vi "Write Coils.vi"(8 "error in (no error)":errorcluster, 9 "values":bool[](array[boolean]), 10 "address":i32, 11 "modbus in":refnum<class "libmodbus.lvclass">) -> (0 "error out":errorcluster, 3 "modbus out":refnum<class "libmodbus.lvclass">)   [LabVIEW 2017, in "libmodbus.lvlib" / "libmodbus.lvclass"]
doc: "Writes single modbus holding register."
uses:
  libmodbus.lvclass
  libmodbus.lvclass/libmodbus.ctl
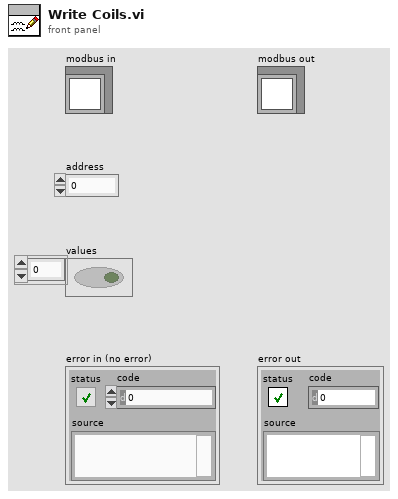
[diagram p1: front panel]
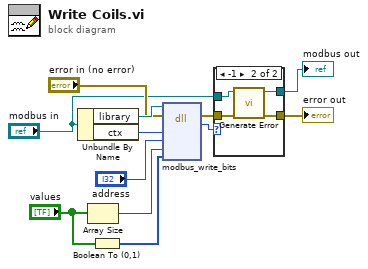
[diagram p0: block diagram]
diagram:
  n1 = Unbundle By Name("modbus in") -> ("library"=w11:path, "ctx"=w12:i64)
  n2 = Array Size(array="values") -> (size(s)=w3:i32)
  n3 = Boolean To (0,1)(Boolean="values") -> (0, 1=w1:i16[])
  n4 = dll-call lib="?" fn="modbus_write_bits"(path in=w11, error in="error in (no error)", "ctx"=w12, "addr"="address", "nb"=w3, "src"=w1) -> (error out=w7:errorcluster, "int"=w9:i32)  [unwired: 5 in, 1 out]
  n5 = case shown="-1" w9 {
    tunnel: [w14 w17] -> w8
    tunnel: w7 -> [w14 w18]
    tunnel: "modbus in" -> [w13 w16]
    tunnel: [w13 w15] -> w5
    frame Default {
    }
    frame -1 {
      n6 = call "Generate Error.vi"("error in (no error)"=w18, "modbus in"=w16) -> ("error out"=w17:errorcluster, "modbus out"=w15:refnum<class "libmodbus.lvclass">)  [unwired: 8 in]
    }
  }
  "modbus out" <- w5
  "error out" <- w8
